vi "Create Test Suite (JUnit).vi.vi"(5 "Interactive (T)":bool=TRUE, 7 "Verbose":bool, 8 "error in (no error)":errorcluster, 11 "Test Runner.JUnit out":refnum<class "Test Runner.JUnit.lvclass">) -> (0 "error out":errorcluster, 3 "Test Runner.JUnit in":refnum<class "Test Runner.JUnit.lvclass">)   [LabVIEW 2013, in "Test Runner.JUnit.lvclass"]
uses:
  Test Runner.JUnit.lvclass
  classes/Test Runner/Test Runner.lvclass/Test Runner.ctl
  classes/Test Runner/Test Runner.lvclass
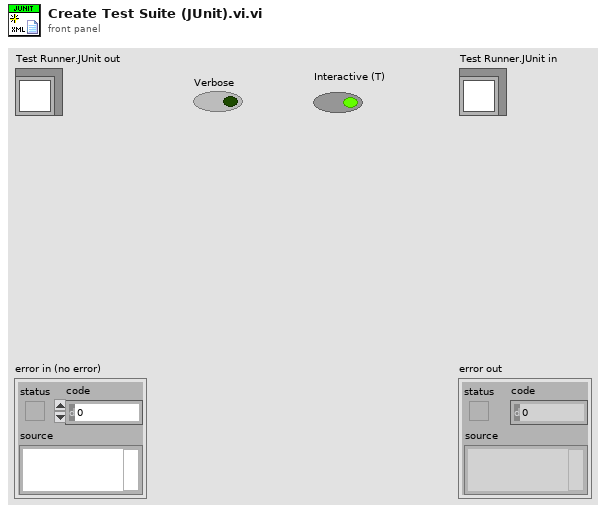
[diagram p1: front panel]
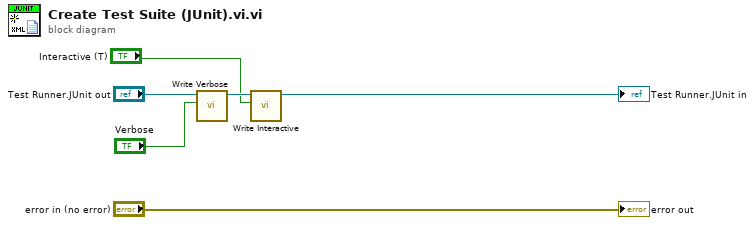
[diagram p0: block diagram]
diagram:
  n1 = call "Write Verbose.vi"("Verbose"="Verbose", "Test Runner in"="Test Runner.JUnit out") -> ("Test Runner out"=w6:refnum<class "Test Runner.JUnit.lvclass">)  [unwired: 9 in]
  n2 = call "Write Interactive.vi"("Interactive"="Interactive (T)", "Test Runner in"=w6) -> ("Test Runner out"=→"Test Runner.JUnit in":refnum<class "Test Runner.JUnit.lvclass">)  [unwired: 9 in]
  "error out" <- "error in (no error)"
